vi "PostTAFMenuHook.vi"(8 "error in (no error)":errorcluster, 10 "MenuIn":T1[](array[typedef]), 11 "MasterGUI in":refnum<class "MasterGUI.lvclass">) -> (0 "error out":errorcluster, 2 "MenuOut":T1[](array[typedef]), 3 "MasterGUI out":refnum<class "MasterGUI.lvclass">)   [LabVIEW 2021, in "MasterGUI.lvclass"]
uses:
  MasterGUI.lvclass
  MenuItem.ctl
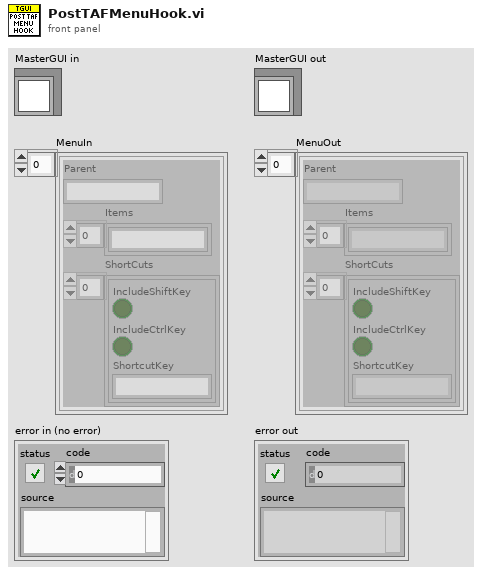
[diagram p1: front panel]
types:
  T1 = typedef "MasterGUI.lvclass/MenuItem.ctl" = cluster{"Parent":string, "Items":string[], "ShortCuts":cluster{"IncludeShiftKey":bool, "IncludeCtrlKey":bool, "ShortcutKey":string}[]}
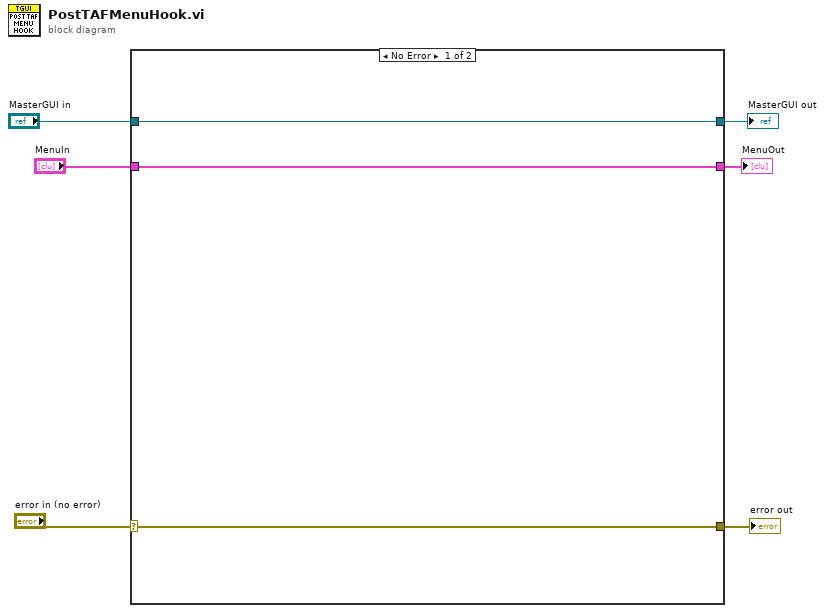
[diagram p0: block diagram]
diagram:
  n1 = case shown="No Error" "error in (no error)" {
    selector: "error in (no error)" -> [w7 w10]
    tunnel: [w7 w10] -> w6
    tunnel: [w8 w11] -> w5
    tunnel: [w9 w12] -> w2
    tunnel: "MasterGUI in" -> [w9 w12]
    tunnel: "MenuIn" -> [w8 w11]
    frame No Error {
    }
    frame Error {
    }
  }
  "MasterGUI out" <- w2
  "error out" <- w6
  "MenuOut" <- w5
